vi "Gaussian Fit with FWHM.vi"(5 "Initial Center":dbl, 7 "Inital Amplitude":dbl, 8 "Gaussian Fit Method":T3 items=["Least Square", "Least Absolute Residual", "Bisquare"], 10 "Y data":dbl[](array[numeric]), 11 "X data":u32[](array[numeric])) -> (0 "error out":errorcluster, 1 "FWHM (X,Y)":cluster{dbl[], dbl[]}, 2 "Gaussian Fit Data":T2, 3 "Gaussian Fit (X,Y)":T1, 4 "Valid Fit?":bool)   [LabVIEW 2012]
uses:
  <vilib>/Analysis/6fits.llb/Curve Fitting Criteria.ctl
  <vilib>/Analysis/NI_AALPro.lvlib
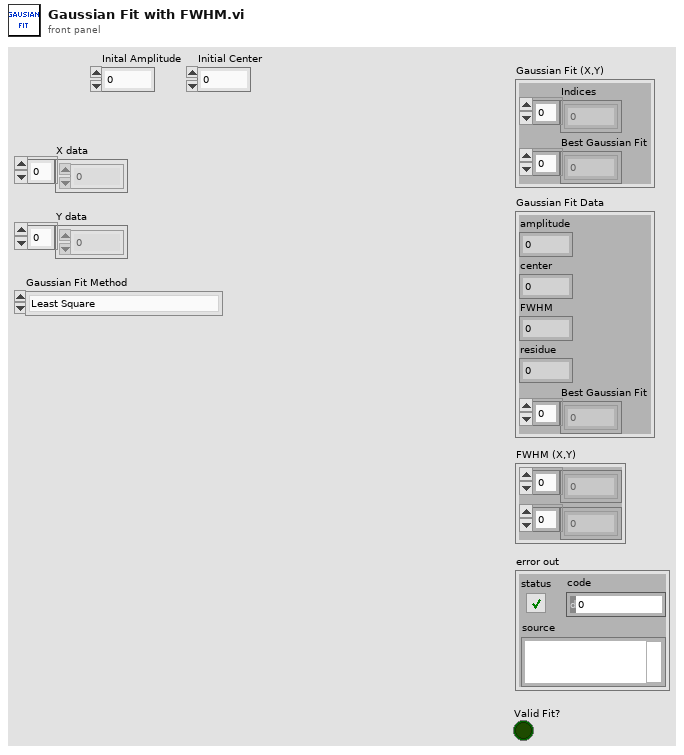
[diagram p1: front panel]
types:
  T1 = cluster{"Indices":u32[], "Best Gaussian Fit":dbl[]}
  T2 = cluster{"amplitude":dbl, "center":dbl, "FWHM":dbl, "residue":dbl, "Best Gaussian Fit":dbl[]}
  T3 = typedef "NI_AALPro.lvlib/Curve Fitting Criteria.ctl" = u16
  T4 = cluster{"initial amplitude":dbl, "initial center":dbl, "initial standard deviation":dbl, "offset":dbl}
  T5 = cluster{"X data":u32[], "Best Gaussian Fit":dbl[]}
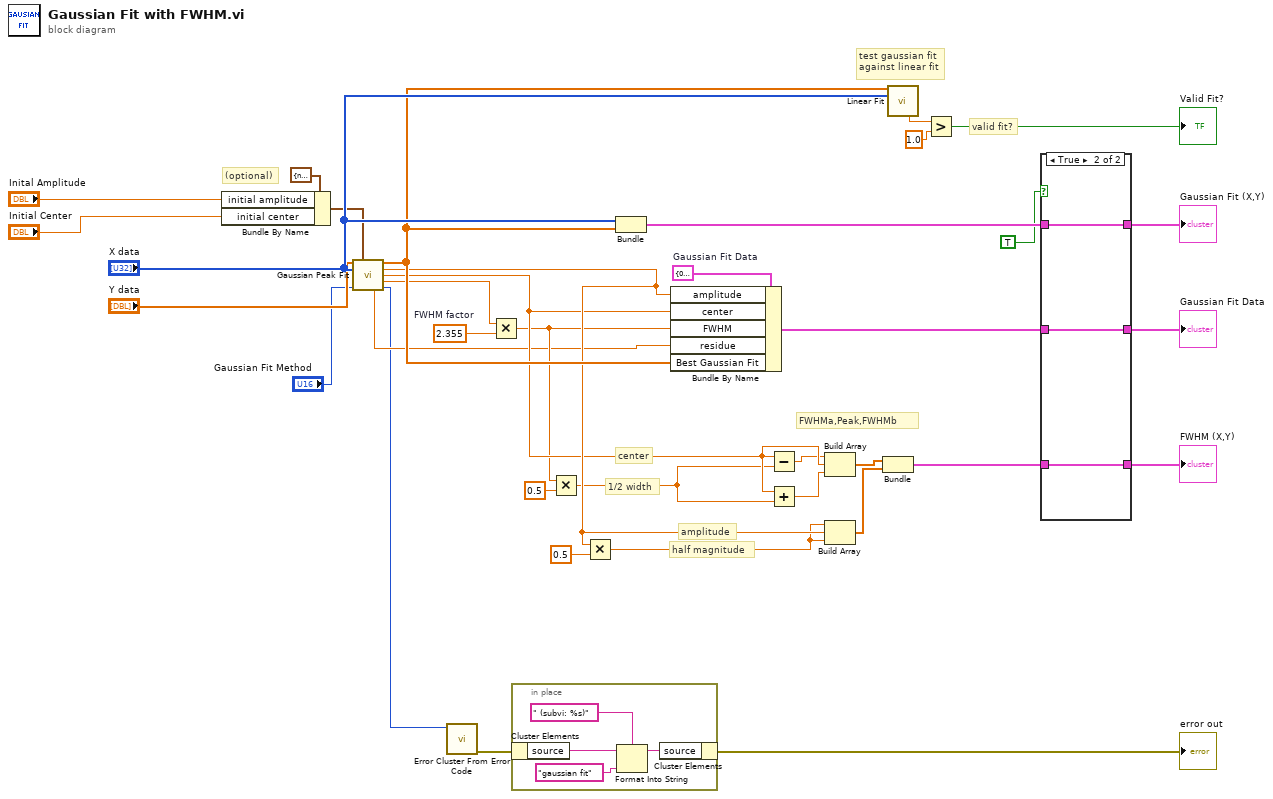
[diagram p0: block diagram]
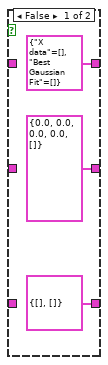
[diagram p2: hidden frame]
diagram:
  w15 = T2 {"amplitude"=0.0, "center"=0.0, "FWHM"=0.0, "residue"=0.0, "Best Gaussian Fit"=[]}  # Gaussian Fit Data
  w13 = 2.355  # FWHM factor
  # "valid fit?"
  # "test gaussian fit\nagainst linear fit"
  # "(optional)"
  # "amplitude"
  # "1/2 width"
  # "FWHMa,Peak,FWHMb"
  # "half magnitude"
  # "center"
  n1 = Bundle By Name(cluster=T4 {"initial amplitude"=nan, "initial center"=nan, "initial standard deviation"=nan, "offset"=nan} ("initial guess"), "initial amplitude"="Inital Amplitude", "initial center"="Initial Center") -> (w30:T4)
  n2 = call <vilib>:"Gaussian Peak Fit.vi"("Y"="Y data", "initial guess"=w30, "X"="X data", "method"="Gaussian Fit Method") -> ("Best Gaussian Fit"=w33:dbl[], "amplitude"=w27:dbl, "center"=w24:dbl, "standard deviation"=w14:dbl, "residue"=w16:dbl, "error"=w10:i32)  [unwired: 5 in, 1 out]
  n3 = call <vilib>:"Error Cluster From Error Code.vi"("error code (0)"=w10) -> ("error out"=w11:errorcluster)  [unwired: 8 in]
  n4 = Multiply(x=w14, y=w13) -> (x*y=w20:dbl)
  n5 = in-place "In Place Element Structure" {
    n6 = in-place-cluster #1(w11) -> ("source"=w38:string)
    n7 = Format Into String(format string=" (subvi: %s)" ("initial string"), initial string=w38, "gaussian fit" ("input 1")) -> (resulting string=w40:string)  [unwired: 1 in, 1 out]
    n8 = in-place-cluster #1("source"=w40) -> (→"error out":errorcluster)
  }
  n9 = Multiply(x=w20, y=0.5) -> (x*y=w22:dbl)
  n10 = Multiply(x=w27, y=0.5) -> (x*y=w26:dbl)
  n11 = Bundle("X data"="X data", "Best Gaussian Fit"=w33) -> (w7:T5)  [unwired: 1 in]
  n12 = Bundle By Name(cluster=w15, "amplitude"=w27, "center"=w24, "FWHM"=w20, "residue"=w16, "Best Gaussian Fit"=w33) -> (w5:T2)
  n13 = Subtract(x=w24, y=w22) -> (x-y=w18:dbl)
  n14 = Add(x=w24, y=w22) -> (x+y=w23:dbl)
  n15 = Build Array(w18, w24, w23) -> (w17:dbl[])
  n16 = Build Array(w26, w27, w26) -> (w19:dbl[])
  n17 = Bundle(w17, w19) -> (w3:cluster{dbl[], dbl[]})  [unwired: 1 in]
  n18 = call <vilib>:"Linear Fit.vi"("Y"=w33, "X"="X data") -> ("residue"=w35:dbl)  [unwired: 9 in, 4 out]
  n19 = Greater?(x=w35, y=1.0) -> (0:→"Valid Fit?":bool)
  n20 = case shown="True" TRUE {
    tunnel: [T5 {"X data"=[], "Best Gaussian Fit"=[]} w46] -> w8
    tunnel: w7 -> [_ w46]
    tunnel: [T2 {"amplitude"=0.0, "center"=0.0, "FWHM"=0.0, "residue"=0.0, "Best Gaussian Fit"=[]} ("Gaussian Fit Data") w45] -> w6
    tunnel: w5 -> [_ w45]
    tunnel: [cluster{dbl[], dbl[]} {[], []} w44] -> w4
    tunnel: w3 -> [_ w44]
    frame False {
    }
    frame True {
    }
  }
  "Gaussian Fit Data" <- w6
  "FWHM (X,Y)" <- w4
  "Gaussian Fit (X,Y)" <- w8
